vi "sv_Convert Variant Attributes to Spectrum Info.vi"(0 "variant attributes":variant, 11 "error in":errorcluster) -> (4 "variant attributes":variant, 10 "spectrum info":T1 {"x-axis units" items=["Time (s)"=0, "Frequency-CB (Hz)"=1, "Frequency-CPB (Hz)"=1248, "Frequency-Arbitrary (Hz)"=2357, "Quefrency (s)"=2, "Revolutions (rev)"=3, "Order"=4, "Speed (RPM)"=11, "Speed (rad/s)"=21, "Index"=65535]; "weighting filter" items=["Linear", "A-weighting", "B-weighting", "C-weighting", "ITU-R 468-4", "Dolby", "CCITT", "C-message", "Wb", "Wc", "Wd", "We", "Wf", "Wh", "Wj", "Wk", "Wm", "AES17 20 kHz lowpass", "AES17 40 kHz lowpass", "AES17 20 kHz highpass", "AES17 40 kHz highpass"]; "dB reference [EU]" format="%.2f"; "engineering units" items=["custom..."=0, "V"=1, "A"=21, "C"=30, "pC"=31, "s"=32, "-"=29, "Pa"=2, "N"=20, "g"=3, "m/s^2"=4, "m/s"=5, "m"=6, "mm/s"=12, "mm"=13, "micron/s"=14, "micron"=15, "in/s^2"=7, "in/s"=8, "in"=9, "mil/s"=10, "mil"=11, "rad/s^2"=16, "rad/s"=17, "rad"=18, "deg/s^2"=26, "deg/s"=27, "deg"=28, "RPM"=22, "cycle/s^2"=23, "Hz"=24, "cycle"=25, "strain"=19]; "spectral info"."window" items=["None "=0, "Hanning"=1, "Hamming"=2, "Blackman-Harris"=3, "Exact Blackman"=4, "Blackman"=5, "Flat Top"=6, "4 Term B-Harris "=7, "7 Term B-Harris"=8, "Low Sidelobe"=9, "Force - Exponential"=10, "Gaussian"=62]}, 15 "error out":errorcluster)   [LabVIEW 2017]
uses:
  <vilib>/addons/_NISVFA/_Shared subVIs/Controls/svc_Spectrum Info.ctl
  <vilib>/addons/_NISVFA/_Shared subVIs/Controls/svc_X-Axis Units.ctl
  <vilib>/addons/_NISVFA/_Shared subVIs/Controls/svc_Spectrum Type.ctl
  <vilib>/addons/_NISVFA/_Shared subVIs/Controls/svc_Engineering Units Text Ring.ctl
  <vilib>/addons/_NISVFA/_Shared subVIs/Controls/svc_Weighting Filter Text Ring.ctl
  <vilib>/addons/_NISVFA/_Shared subVIs/Controls/svc_Complimentary Spectrum Units.ctl
  <vilib>/addons/_NISVFA/_Shared subVIs/Controls/NI Channel Properties.ctl
  <vilib>/addons/_NISVFA/_Shared subVIs/Controls/NI Function Type.ctl
  <vilib>/addons/_NISVFA/_Shared subVIs/Controls/NI Function SubType.ctl
  <vilib>/addons/_NISVFA/_Shared subVIs/Controls/LV Datatypes.ctl
  <vilib>/addons/_NISVFA/_Shared subVIs/Controls/SV Channel Properties.ctl
  <vilib>/addons/_NISVFA/_Shared subVIs/Common/svc_Get Weighting Enum and Labels.vi
  <vilib>/addons/_NISVFA/_Shared subVIs/Common/svc_Unit Label Lexical Class.vi
  <vilib>/addons/_NISVFA/_Shared subVIs/Common/svc_Format Value (DBL).vi
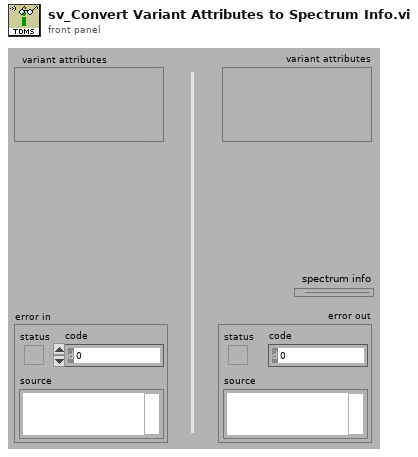
[diagram p1: front panel]
types:
  T1 = typedef "svc_Spectrum Info.ctl" = cluster{"channel name":string, "description":string, "x-axis units":T2, "spectral info":cluster{"spectrum type":T3, "linear/dB":enum16{"linear", "dB"}, "window":u16, "window size":i32, "FFT size":i32}, "engineering units":T4, "custom label":string, "dB reference [EU]":dbl, "peak units":enum16{"rms", "peak", "peak-peak"}, "weighting filter":T5, "spectral density?":bool, "unit label":string, "spectrum skewed?":bool, "complimentary spectrum units":T6}
  T2 = typedef "svc_X-Axis Units.ctl" = u16
  T3 = typedef "svc_Spectrum Type.ctl" = enum16{"FFT Spectrum [complex]", "Amplitude [Magnitude]", "Power [Magnitude^2]", "Cross Spectrum [complex]", "Frequency Response [Complex]"}
  T4 = typedef "svc_Engineering Units Text Ring.ctl" = u16
  T5 = typedef "svc_Weighting Filter Text Ring.ctl" = u16
  T6 = typedef "svc_Complimentary Spectrum Units.ctl" = enum16{"none", "radians", "degrees", "cycles", "imaginary"}
  T7 = typedef "SV Channel Properties.ctl" = u16
  T8 = typedef "NI Channel Properties.ctl" = u16
  T9 = typedef "LV Datatypes.ctl" = i32
  T10 = typedef "NI Function Type.ctl" = u16
  T11 = typedef "NI Function SubType.ctl" = u16
  T12 = cluster{"function type":T10, "function subtype":T11, "X-dimension":T2}
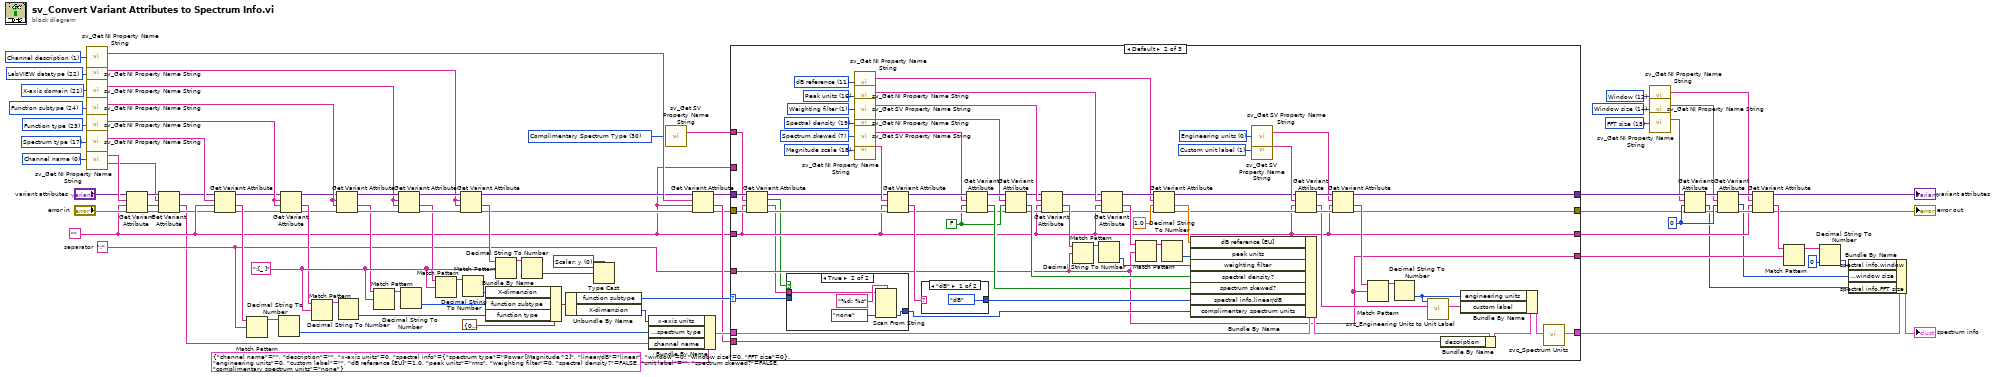
[diagram p0: block diagram]
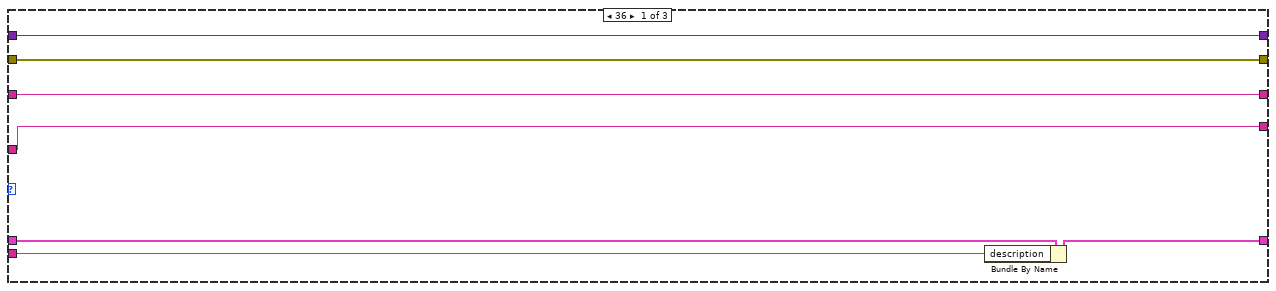
[diagram p2: hidden frame]
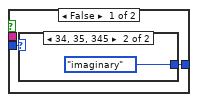
[diagram p3: hidden frame]
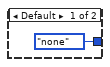
[diagram p4: hidden frame]
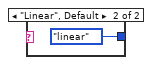
[diagram p5: hidden frame]
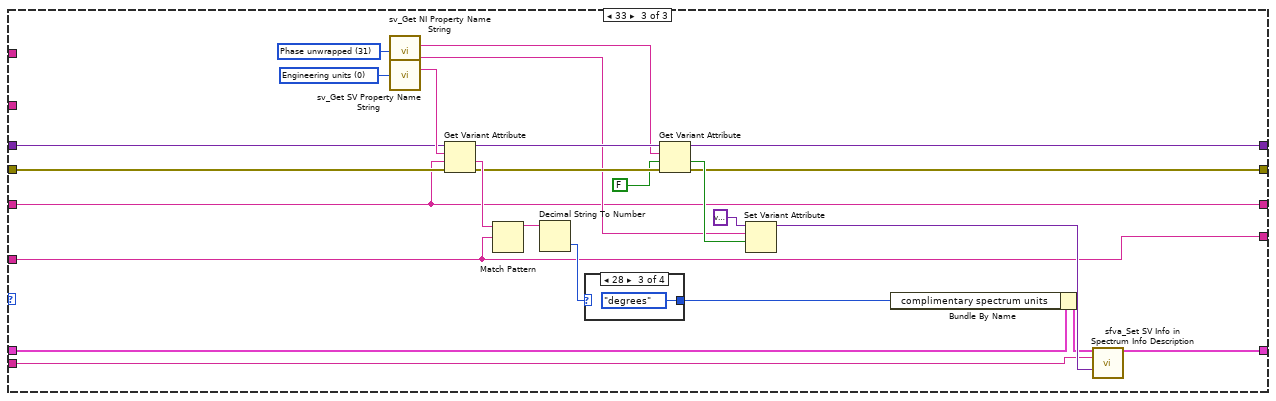
[diagram p6: hidden frame]
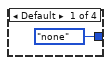
[diagram p7: hidden frame]
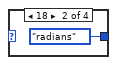
[diagram p8: hidden frame]
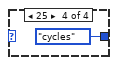
[diagram p9: hidden frame]
diagram:
  w9 = T7 30 items=["Engineering units", "Custom unit label", "Weighting filter", "Pregain", "Octave standard", "Octave bandwidth", "Octave low band", "Octave high band", "Spectrum skewed", "Samples / revolution", "Order", "Tachometer", "Pulses Per Revolution", "Rotation Direction", "Probe Angle", "Pair", "Channel Alias", "Tachometer Threshold", "Tachometer Slope", "Max Order", "Sensor Location", "Sensor Orientation", "Analog Software Trigger", "Trigger Level", "Pretrigger Samples", "Trigger Slope", "Trigger Hysteresis", "Sensor sensitivity", "Sensor type", "Sensor maximum", "Complimentary Spectrum Type"] ("property")
  w29 = T8 15 items=["Channel name", "Channel description", "Y-axis label", "Y-axis unit string", "X-axis label", "X-axis unit string", "x0", "dx", "Number of samples", "X channel", "Filter settled", "dB reference", "Window", "Window parameter", "Window size", "FFT size", "Peak units", "Spectrum type", "Magnitude scale", "Spectral density"] ("property")
  w28 = T8 14 items=["Channel name", "Channel description", "Y-axis label", "Y-axis unit string", "X-axis label", "X-axis unit string", "x0", "dx", "Number of samples", "X channel", "Filter settled", "dB reference", "Window", "Window parameter", "Window size", "FFT size", "Peak units", "Spectrum type", "Magnitude scale", "Spectral density"] ("property")
  w27 = T8 12 items=["Channel name", "Channel description", "Y-axis label", "Y-axis unit string", "X-axis label", "X-axis unit string", "x0", "dx", "Number of samples", "X channel", "Filter settled", "dB reference", "Window", "Window parameter", "Window size", "FFT size", "Peak units", "Spectrum type", "Magnitude scale", "Spectral density"] ("property")
  w34 = 0 ("FFT size")
  w45 = T8 0 items=["Channel name", "Channel description", "Axis label", "Unit string", "Waveform X-axis label", "Waveform X-axis unit string", "x0", "dx", "Number of samples", "X channel", "Filter settled", "dB reference", "Window", "Window parameter", "Window size", "FFT size", "Peak units", "Spectrum type", "Magnitude scale", "Spectral density", "Sensor sensitivity (mV/EU)", "X-axis dimension", "LabVIEW datatype", "Function type", "Function subtype", "X values", "Independent channel", "Column index", "Collection name", "Collection ID", "X Columns", "Phase unwrapped"] ("property")
  w50 = T9 0 items=["String: abc"=7, "Boolean: True or False"=8, "Scalar: y"=0, "Array: Y"=1, "Waveform: t0, dt, Y, variant"=2, "Cluster: x0, dx, Y"=3, "Cluster: X, Y"=4, "Waterfall"=5, "Colormap"=6] ("LabVIEW datatype")
  w70 = ":[_ ]" ("regular expression")
  w69 = T8 22 items=["Channel name", "Channel description", "Y-axis label", "Y-axis unit string", "X-axis label", "X-axis unit string", "x0", "dx", "Number of samples", "X channel", "Filter settled", "dB reference", "Window", "Window parameter", "Window size", "FFT size", "Peak units", "Spectrum type", "Magnitude scale", "Spectral density", "Sensor sensitivity (mV/EU)", "X-axis domain", "LabVIEW datatype"] ("property")
  w67 = T8 24 items=["Channel name", "Channel description", "Y-axis label", "Y-axis unit string", "X-axis label", "X-axis unit string", "x0", "dx", "Number of samples", "X channel", "Filter settled", "dB reference", "Window", "Window parameter", "Window size", "FFT size", "Peak units", "Spectrum type", "Magnitude scale", "Spectral density", "Sensor sensitivity (mV/EU)", "X-axis dimension", "LabVIEW datatype", "Function type", "Function subtype"] ("property")
  w68 = T8 21 items=["Channel name", "Channel description", "Y-axis label", "Y-axis unit string", "X-axis label", "X-axis unit string", "x0", "dx", "Number of samples", "X channel", "Filter settled", "dB reference", "Window", "Window parameter", "Window size", "FFT size", "Peak units", "Spectrum type", "Magnitude scale", "Spectral density", "Sensor sensitivity (mV/EU)", "X-axis domain", "LabVIEW datatype", "Function type", "Component", "Level detector"] ("property")
  w66 = T8 23 items=["Channel name", "Channel description", "Y-axis label", "Y-axis unit string", "X-axis label", "X-axis unit string", "x0", "dx", "Number of samples", "X channel", "Filter settled", "dB reference", "Window", "Window parameter", "Window size", "FFT size", "Peak units", "Spectrum type", "Magnitude scale", "Spectral density", "Sensor sensitivity (mV/EU)", "X-axis domain", "LabVIEW datatype", "Function type", "Component", "Level detector"] ("property")
  w82 = T8 1 items=["Channel name", "Channel description", "Axis label", "Unit string", "Waveform X-axis label", "Waveform X-axis unit string", "x0", "dx", "Number of samples", "X channel", "Filter settled", "dB reference", "Window", "Window parameter", "Window size", "FFT size", "Peak units", "Spectrum type", "Magnitude scale", "Spectral density", "Sensor sensitivity (mV/EU)", "X-axis dimension", "LabVIEW datatype", "Function type", "Function subtype", "X values", "Independent channel", "Column index", "Collection name", "Collection ID", "X Columns", "Phase unwrapped"] ("property")
  w37 = ":"  # separator
  w36 = "" ("TDMS property name")
  w88 = T8 17 items=["Channel name", "Channel description", "Y-axis label", "Y-axis unit string", "X-axis label", "X-axis unit string", "x0", "dx", "Number of samples", "X channel", "Filter settled", "dB reference", "Window", "Window parameter", "Window size", "FFT size", "Peak units", "Spectrum type", "Magnitude scale", "Spectral density"] ("property")
  n1 = call <vilib>:"sv_Get NI Property Name String.vi"("property"=w82) -> ("TDMS property name"=w48:string)  [unwired: 13 in, 1 out]
  n2 = call <vilib>:"sv_Get NI Property Name String.vi"("property"=w69) -> ("TDMS property name"=w53:string)  [unwired: 13 in, 1 out]
  n3 = call <vilib>:"sv_Get NI Property Name String.vi"("property"=w68) -> ("TDMS property name"=w57:string)  [unwired: 13 in, 1 out]
  n4 = call <vilib>:"sv_Get NI Property Name String.vi"("property"=w67) -> ("TDMS property name"=w63:string)  [unwired: 13 in, 1 out]
  n5 = call <vilib>:"sv_Get NI Property Name String.vi"("property"=w66) -> ("TDMS property name"=w65:string)  [unwired: 13 in, 1 out]
  n6 = call <vilib>:"sv_Get NI Property Name String.vi"("property"=w88) -> ("TDMS property name"=w80:string)  [unwired: 13 in, 1 out]
  n7 = call <vilib>:"sv_Get NI Property Name String.vi"("property"=w45) -> ("TDMS property name"=w44:string, "WDT attribute name"=w2:string)  [unwired: 13 in]
  n8 = Get Variant Attribute(Variant="variant attributes", name=w44, default value (empty Variant)=w36, error in="error in") -> (duplicate Variant=w5:variant, value=w6:string, error out=w7:errorcluster)  [unwired: 1 out]
  n9 = Get Variant Attribute(Variant=w5, name=w2, default value (empty Variant)=w6, error in=w7) -> (duplicate Variant=w3:variant, value=w1:string, error out=w4:errorcluster)  [unwired: 1 out]
  n10 = Get Variant Attribute(Variant=w3, name=w80, default value (empty Variant)=w36, error in=w4) -> (duplicate Variant=w46:variant, value=w79:string, error out=w39:errorcluster)  [unwired: 1 out]
  n11 = Match Pattern(string=w79, regular expression=w37) -> (before substring=w87:string)  [unwired: 1 in, 3 out]
  n12 = Decimal String To Number(string=w87) -> (number=w86:i32)  [unwired: 2 in, 1 out]
  n13 = Get Variant Attribute(Variant=w46, name=w65, default value (empty Variant)=w65, error in=w39) -> (duplicate Variant=w62:variant, value=w64:string, error out=w61:errorcluster)  [unwired: 1 out]
  n14 = Match Pattern(string=w64, regular expression=w70) -> (before substring=w78:string)  [unwired: 1 in, 3 out]
  n15 = Get Variant Attribute(Variant=w62, name=w63, default value (empty Variant)=w63, error in=w61) -> (duplicate Variant=w58:variant, value=w59:string, error out=w60:errorcluster)  [unwired: 1 out]
  n16 = Decimal String To Number(string=w78) -> (number=w76:i32)  [unwired: 2 in, 1 out]
  n17 = Match Pattern(string=w59, regular expression=w70) -> (before substring=w75:string)  [unwired: 1 in, 3 out]
  n18 = Get Variant Attribute(Variant=w58, name=w57, default value (empty Variant)=w57, error in=w60) -> (duplicate Variant=w54:variant, value=w55:string, error out=w56:errorcluster)  [unwired: 1 out]
  n19 = Decimal String To Number(string=w75) -> (number=w74:i32)  [unwired: 2 in, 1 out]
  n20 = Match Pattern(string=w55, regular expression=w70) -> (before substring=w71:string)  [unwired: 1 in, 3 out]
  n21 = Get Variant Attribute(Variant=w54, name=w53, default value (empty Variant)=w53, error in=w56) -> (duplicate Variant=w41:variant, value=w52:string, error out=w40:errorcluster)  [unwired: 1 out]
  n22 = Decimal String To Number(string=w71) -> (number=w73:i32)  [unwired: 2 in, 1 out]
  n23 = Bundle By Name(cluster=T12 {"function type"=0, "function subtype"=0, "X-dimension"=0} ("function info"), "X-dimension"=w73, "function subtype"=w74, "function type"=w76) -> (w51:T12)
  n24 = Match Pattern(string=w52, regular expression=w70) -> (before substring=w72:string)  [unwired: 1 in, 3 out]
  n25 = Decimal String To Number(string=w72) -> (number=w49:i32)  [unwired: 2 in, 1 out]
  n26 = Unbundle By Name(w51) -> ("function subtype"=w84:T11, "X-dimension"=w83:T2)
  n27 = Type Cast(type=w50, x=w49) -> ()  [unwired: 1 out]
  n28 = Bundle By Name(cluster=T1 {"channel name"="", "description"="", "x-axis units"=0, "spectral info"={"spectrum type"=enum."Power [Magnitude^2]", "linear/dB"=enum."linear", "window"=0, "window size"=0, "FFT size"=0}, "engineering units"=0, "custom label"="", "dB reference [EU]"=1.0, "peak units"=enum."rms", "weighting filter"=0, "spectral density?"=FALSE, "unit label"="", "spectrum skewed?"=FALSE, "complimentary spectrum units"=enum."none"} ("spectrum info in"), "x-axis units"=w83, "spectral info.spectrum type"=w86, "channel name"=w1) -> (w85:T1)
  n29 = call <vilib>:"sv_Get SV Property Name String.vi"("property"=w9) -> ("TDMS property name"=w8:string)  [unwired: 13 in, 1 out]
  n30 = Get Variant Attribute(Variant=w41, name=w48, default value (empty Variant)=w36, error in=w40) -> (duplicate Variant=w35:variant, value=w47:string, error out=w38:errorcluster)  [unwired: 1 out]
  n31 = case shown="Default" w84 {
    selector: w84 -> [_ w140 _]
    tunnel: [w89 w105 w177] -> w17
    tunnel: [w95 w106 w176] -> w18
    tunnel: w38 -> [w95 w100 w183]
    tunnel: w36 -> [_ _ _]
    tunnel: w37 -> [w90 w104 w173]
    tunnel: w85 -> [w94 w149 w195]
    tunnel: [w93 w146 w189] -> w20
    tunnel: w47 -> [w92 w141 w188]
    tunnel: w36 -> [w91 w98 w174]
    tunnel: w35 -> [w89 w103 w184]
    tunnel: [w90 w104 w173] -> w25
    tunnel: [w91 w98 w174] -> w24
    tunnel: w8 -> [_ w101 _]
    frame 36 {
      n32 = Bundle By Name(cluster=w94, "description"=w92) -> (w93:T1)
    }
    frame Default {
      w130 = FALSE ("spectrum skewed?")
      w155 = T8 18 items=["Channel name", "Channel description", "Y-axis label", "Y-axis unit string", "X-axis label", "X-axis unit string", "x0", "dx", "Number of samples", "X channel", "Filter settled", "dB reference", "Window", "Window parameter", "Window size", "FFT size", "Peak units", "Spectrum type", "Magnitude scale", "Spectral density"] ("property")
      w156 = T7 0 items=["Engineering units", "Weighting filter", "Pregain", "Octave standard", "Octave bandwidth", "Octave low band", "Octave high band", "Spectrum skewed"] ("property")
      w157 = T7 1 items=["Engineering units", "Custom unit label", "Weighting filter", "Pregain", "Octave standard", "Octave bandwidth", "Octave low band", "Octave high band", "Spectrum skewed"] ("property")
      w158 = T8 11 items=["Channel name", "Channel description", "Y-axis label", "Y-axis unit string", "X-axis label", "X-axis unit string", "x0", "dx", "Number of samples", "X channel", "Filter settled", "dB reference", "Window", "Window parameter", "Window size", "FFT size", "Peak units", "Spectrum type", "Magnitude scale", "Spectral density"] ("property")
      w159 = T8 16 items=["Channel name", "Channel description", "Y-axis label", "Y-axis unit string", "X-axis label", "X-axis unit string", "x0", "dx", "Number of samples", "X channel", "Filter settled", "dB reference", "Window", "Window parameter", "Window size", "FFT size", "Peak units", "Spectrum type", "Magnitude scale", "Spectral density"] ("property")
      w160 = T8 19 items=["Channel name", "Channel description", "Y-axis label", "Y-axis unit string", "X-axis label", "X-axis unit string", "x0", "dx", "Number of samples", "X channel", "Filter settled", "dB reference", "Window", "Window parameter", "Window size", "FFT size", "Peak units", "Spectrum type", "Magnitude scale", "Spectral density"] ("property")
      w161 = T7 7 items=["Engineering units", "Weighting filter", "Pregain", "Octave standard", "Octave bandwidth", "Octave low band", "Octave high band", "Spectrum skewed"] ("property")
      w162 = T7 1 items=["Engineering units", "Weighting filter", "Pregain", "Octave standard", "Octave bandwidth", "Octave low band", "Octave high band", "Spectrum skewed"] ("property")
      n33 = Get Variant Attribute(Variant=w103, name=w101, default value (empty Variant)=w98, error in=w100) -> (duplicate Variant=w102:variant, found=w97:bool, value=w96:string, error out=w99:errorcluster)
      n34 = case shown="True" w97 {
        tunnel: w140 -> [w164 _]
        tunnel: [w163 w169] -> w139
        tunnel: w96 -> [_ w167]
        frame False {
          n35 = case shown="34, 35, 345" w164 {
            tunnel: [svc_Complimentary_Spectrum_Units."none" ("complimentary spectrum units") svc_Complimentary_Spectrum_Units."imaginary" ("complimentary spectrum units")] -> w163
            frame Default {
            }
            frame 34, 35, 345 {
            }
          }
        }
        frame True {
          n36 = Scan From String(format string="%d: %s", input string=w167, default 2=svc_Complimentary_Spectrum_Units."none" ("complimentary spectrum units 2")) -> (output 2=w169:T6)  [unwired: 4 in, 3 out]
        }
      }
      n37 = call <vilib>:"sv_Get NI Property Name String.vi"("property"=w158) -> ("TDMS property name"=w118:string)  [unwired: 13 in, 1 out]
      n38 = call <vilib>:"sv_Get NI Property Name String.vi"("property"=w159) -> ("TDMS property name"=w123:string)  [unwired: 13 in, 1 out]
      n39 = call <vilib>:"sv_Get SV Property Name String.vi"("property"=w162) -> ("TDMS property name"=w127:string)  [unwired: 13 in, 1 out]
      n40 = call <vilib>:"sv_Get NI Property Name String.vi"("property"=w160) -> ("TDMS property name"=w131:string)  [unwired: 13 in, 1 out]
      n41 = call <vilib>:"sv_Get SV Property Name String.vi"("property"=w161) -> ("TDMS property name"=w135:string)  [unwired: 13 in, 1 out]
      n42 = call <vilib>:"sv_Get NI Property Name String.vi"("property"=w155) -> ("TDMS property name"=w138:string)  [unwired: 13 in, 1 out]
      n43 = Get Variant Attribute(Variant=w102, name=w138, default value (empty Variant)=w98, error in=w99) -> (duplicate Variant=w136:variant, value=w137:string, error out=w134:errorcluster)  [unwired: 1 out]
      n44 = case shown="\"dB\"" w137 {
        tunnel: [enum16{"linear", "dB"}."dB" ("spectral info.linear/dB") enum16{"linear", "dB"}."linear" ("spectral info.linear/dB")] -> w154
        frame "dB" {
        }
        frame "Linear", Default {
        }
      }
      n45 = Get Variant Attribute(Variant=w136, name=w135, default value (empty Variant)=w130, error in=w134) -> (duplicate Variant=w132:variant, value=w133:bool, error out=w128:errorcluster)  [unwired: 1 out]
      n46 = Get Variant Attribute(Variant=w132, name=w131, default value (empty Variant)=w130, error in=w128) -> (duplicate Variant=w126:variant, value=w129:bool, error out=w125:errorcluster)  [unwired: 1 out]
      n47 = Get Variant Attribute(Variant=w126, name=w127, default value (empty Variant)=w98, error in=w125) -> (duplicate Variant=w122:variant, value=w124:string, error out=w121:errorcluster)  [unwired: 1 out]
      n48 = Match Pattern(string=w124, regular expression=w104) -> (before substring=w153:string)  [unwired: 1 in, 3 out]
      n49 = Decimal String To Number(string=w153) -> (number=w150:i32)  [unwired: 2 in, 1 out]
      n50 = Get Variant Attribute(Variant=w122, name=w123, default value (empty Variant)=w98, error in=w121) -> (duplicate Variant=w119:variant, value=w120:string, error out=w115:errorcluster)  [unwired: 1 out]
      n51 = Match Pattern(string=w120, regular expression=w104) -> (before substring=w152:string)  [unwired: 1 in, 3 out]
      n52 = Get Variant Attribute(Variant=w119, name=w118, default value (empty Variant)=1.0 ("x"), error in=w115) -> (duplicate Variant=w111:variant, value=w116:dbl, error out=w107:errorcluster)  [unwired: 1 out]
      n53 = Decimal String To Number(string=w152) -> (number=w151:i32)  [unwired: 2 in, 1 out]
      n54 = Bundle By Name(cluster=w149, "dB reference [EU]"=w116, "peak units"=w151, "weighting filter"=w150, "spectral density?"=w129, "spectrum skewed?"=w133, "spectral info.linear/dB"=w154, "complimentary spectrum units"=w139) -> (w143:T1)
      n55 = call <vilib>:"sv_Get SV Property Name String.vi"("property"=w156) -> ("TDMS property name"=w110:string)  [unwired: 13 in, 1 out]
      n56 = call <vilib>:"sv_Get SV Property Name String.vi"("property"=w157) -> ("TDMS property name"=w112:string)  [unwired: 13 in, 1 out]
      n57 = Get Variant Attribute(Variant=w111, name=w112, default value (empty Variant)=w98, error in=w107) -> (duplicate Variant=w113:variant, value=w108:string, error out=w114:errorcluster)  [unwired: 1 out]
      n58 = Get Variant Attribute(Variant=w113, name=w110, default value (empty Variant)=w98, error in=w114) -> (duplicate Variant=w105:variant, value=w109:string, error out=w106:errorcluster)  [unwired: 1 out]
      n59 = Match Pattern(string=w109, regular expression=w104) -> (before substring=w148:string)  [unwired: 1 in, 3 out]
      n60 = Decimal String To Number(string=w148) -> (number=w145:i32)  [unwired: 2 in, 1 out]
      n61 = call <vilib>:"svc_Engineering Units to Unit Label.vi"("custom label"=w108, "engineering units"=w145) -> ("unit label"=w144:string)  [unwired: 8 in, 1 out]
      n62 = Bundle By Name(cluster=w143, "description"=w141) -> (w142:T1)
      n63 = Bundle By Name(cluster=w142, "engineering units"=w145, "custom label"=w144) -> (w147:T1)
      n64 = call <vilib>:"svc_Spectrum Units.vi"("spectrum info in"=w147) -> ("spectrum info out"=w146:T1)  [unwired: 3 in, 3 out]
    }
    frame 33 {
      w192 = T8 31 items=["Channel name", "Channel description", "Axis label", "Unit string", "Waveform X-axis label", "Waveform X-axis unit string", "x0", "dx", "Number of samples", "X channel", "Filter settled", "dB reference", "Window", "Window parameter", "Window size", "FFT size", "Peak units", "Spectrum type", "Magnitude scale", "Spectral density", "Sensor sensitivity (mV/EU)", "X-axis dimension", "LabVIEW datatype", "Function type", "Function subtype", "X values", "Independent channel", "Column index", "Collection name", "Collection ID", "X Columns", "Phase unwrapped"] ("property")
      w197 = T7 0 items=["Engineering units", "Custom unit label", "Weighting filter", "Pregain", "Octave standard", "Octave bandwidth", "Octave low band", "Octave high band", "Spectrum skewed"] ("SV property")
      n65 = call <vilib>:"sv_Get NI Property Name String.vi"("property"=w192) -> ("TDMS property name"=w179:string, "WDT attribute name"=w175:string)  [unwired: 13 in]
      n66 = call <vilib>:"sv_Get SV Property Name String.vi"("property"=w197) -> ("TDMS property name"=w186:string)  [unwired: 13 in, 1 out]
      n67 = Get Variant Attribute(Variant=w184, name=w186, default value (empty Variant)=w174, error in=w183) -> (duplicate Variant=w182:variant, value=w185:string, error out=w181:errorcluster)  [unwired: 1 out]
      n68 = Match Pattern(string=w185, regular expression=w173) -> (before substring=w196:string)  [unwired: 1 in, 3 out]
      n69 = Decimal String To Number(string=w196) -> (number=w194:i32)  [unwired: 2 in, 1 out]
      n70 = case shown="28" w194 {
        tunnel: [svc_Complimentary_Spectrum_Units."none" ("complimentary spectrum units") svc_Complimentary_Spectrum_Units."radians" ("complimentary spectrum units") svc_Complimentary_Spectrum_Units."degrees" ("complimentary spectrum units") svc_Complimentary_Spectrum_Units."cycles" ("complimentary spectrum units")] -> w193
        frame Default {
        }
        frame 18 {
        }
        frame 28 {
        }
        frame 25 {
        }
      }
      n71 = Get Variant Attribute(Variant=w182, name=w179, default value (empty Variant)=FALSE ("spectrum skewed?"), error in=w181) -> (duplicate Variant=w177:variant, value=w178:bool, error out=w176:errorcluster)  [unwired: 1 out]
      n72 = Set Variant Attribute(Variant=variant ("variant"), name=w175, value=w178) -> (Variant out=w191:variant)  [unwired: 1 in, 2 out]
      n73 = Bundle By Name(cluster=w195, "complimentary spectrum units"=w193) -> (w190:T1)
      n74 = call <vilib>:"sfva_Set SV Info in Spectrum Info Description.vi"("spectrum info"=w190, "description"=w188, "SV Info"=w191) -> ("spectrum info"=w189:T1)  [unwired: 11 in, 1 out]
    }
  }
  n75 = call <vilib>:"sv_Get NI Property Name String.vi"("property"=w27) -> ("TDMS property name"=w12:string)  [unwired: 13 in, 1 out]
  n76 = call <vilib>:"sv_Get NI Property Name String.vi"("property"=w28) -> ("TDMS property name"=w13:string)  [unwired: 13 in, 1 out]
  n77 = call <vilib>:"sv_Get NI Property Name String.vi"("property"=w29) -> ("TDMS property name"=w14:string)  [unwired: 13 in, 1 out]
  n78 = Get Variant Attribute(Variant=w17, name=w14, default value (empty Variant)=w34, error in=w18) -> (duplicate Variant=w31:variant, value=w21:i32, error out=w30:errorcluster)  [unwired: 1 out]
  n79 = Get Variant Attribute(Variant=w31, name=w13, default value (empty Variant)=w34, error in=w30) -> (duplicate Variant=w32:variant, value=w22:i32, error out=w33:errorcluster)  [unwired: 1 out]
  n80 = Get Variant Attribute(Variant=w32, name=w12, default value (empty Variant)=w24, error in=w33) -> (duplicate Variant=→"variant attributes":variant, value=w23:string, error out=→"error out":errorcluster)  [unwired: 1 out]
  n81 = Match Pattern(string=w23, regular expression=w25) -> (before substring=w26:string)  [unwired: 1 in, 3 out]
  n82 = Decimal String To Number(string=w26, default (0L)=u16 0 ("spectral info.window")) -> (number=w11:u16)  [unwired: 1 in, 1 out]
  n83 = Bundle By Name(cluster=w20, "spectral info.window"=w11, "spectral info.window size"=w22, "spectral info.FFT size"=w21) -> (→"spectrum info":T1)
